vi "Key Up.vi"(8 "error in (no error)":errorcluster, 10 "delay in ms (20)":u32=20, 11 "Virtual Key":u8(ring)=65) -> (0 "error out":errorcluster)   [LabVIEW 2023]
doc: "Call the keybd_event function in user32.dll to generate an event corresponding to the key up action\nfor the desired key"
uses:
  03aa9192-3ecb-4dc8-b085-152dd0dc2f43.vi
  User32.dll
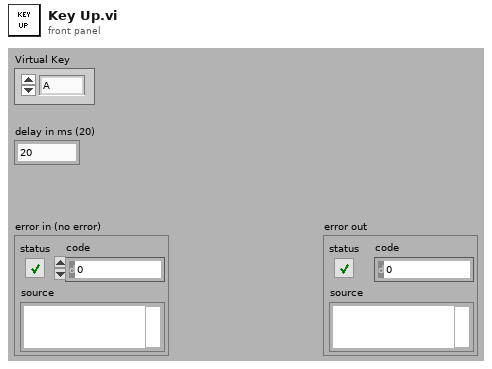
[diagram p1: front panel]
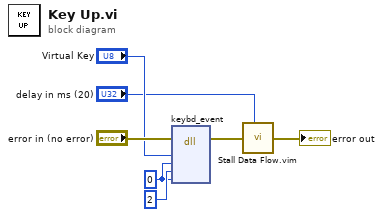
[diagram p0: block diagram]
diagram:
  w5 = u8 0 ("bScan")
  n1 = dll-call lib="user32.dll" fn="keybd_event"(error in="error in (no error)", "bVk"="Virtual Key", "bScan"=w5, "dwFlags"=u32 2, "dwExtraInfo"=w5) -> (error out=w2:errorcluster)  [unwired: 7 in, 1 out]
  n2 = call "Stall Data Flow.vim"("value in"=w2, "milliseconds to wait"="delay in ms (20)") -> ("value out"=→"error out":errorcluster)  [unwired: 1 out]
